vi "ConfigAcquisition.vi"(8 "error in (no error)":errorcluster, 11 "IVI_Class in":refnum<class "IVI_Class.lvclass">) -> (0 "error out":errorcluster, 3 "IVI_Class out":refnum<class "IVI_Class.lvclass">)   [LabVIEW 2018, in "ScopePlugins.lvlib" / "IVI_Class.lvclass"]
uses:
  IVI_Class.lvclass
  C:/Users/ico/Documents/Projects/NistPluggableModules/Scope/ScopePlugins/ScopePluginBaseClass/ScopePluginsBase.lvclass
  ScopePluginBaseClass/ScopePluginsBase.lvclass/ScopePluginsBase.ctl
  ScopePluginBaseClass/Accessors/Read Connected.vi
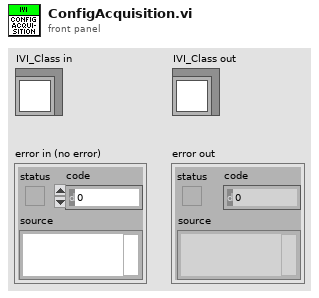
[diagram p1: front panel]
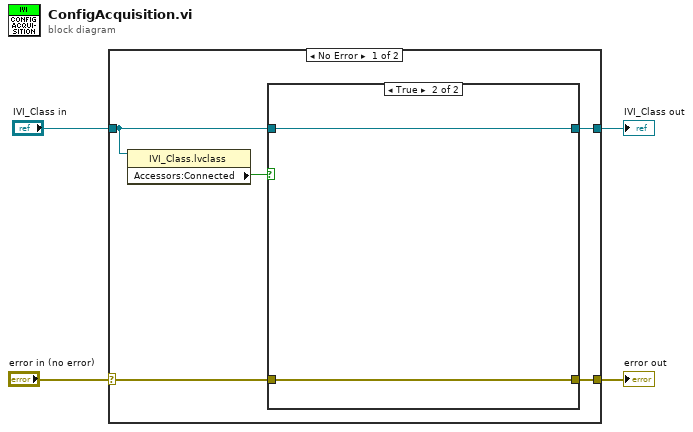
[diagram p0: block diagram]
diagram:
  n1 = case shown="No Error" "error in (no error)" {
    selector: "error in (no error)" -> [w6 w15]
    tunnel: [w7 w14] -> w2
    tunnel: "IVI_Class in" -> [w8 w14]
    tunnel: [w5 w15] -> w1
    frame No Error {
      n2 = property class="IVI_Class.lvclass"(reference=w8) -> ("Accessors:Connected"=w9:bool)  [unwired: 1 in, 2 out]
      n3 = case shown="True" w9 {
        tunnel: w8 -> [w11 w13]
        tunnel: [w11 w13] -> w7
        tunnel: [w10 w12] -> w5
        tunnel: w6 -> [w10 w12]
        frame False {
        }
        frame True {
        }
      }
    }
    frame Error {
    }
  }
  "error out" <- w1
  "IVI_Class out" <- w2
